vi "NIIE_Settings Init.vi"(7 "Refs":T8, 8 "Error":errorcluster, 10 "Active Tag":string="Icon Editor", 11 "Data In":T1={"Class"={"Ants"=refnum, "Layer"=refnum, "Templates"=refnum, "Icon"=refnum, "Glyph"=refnum, "Settings"=refnum, "Tools"=refnum}, "Ref"={"Add Layer"=refnum, "Remove Layer"=refnum, "Line Text"=[], "Body Text Spec"=refnum, "DNL_Font"=refnum, "glyph path str"=refnum, "templates path str"=refnum, "Arrow Up"=refnum, "Arrow Down"=refnum, "IE VI Ref"=refnum, "Glyphs tree"=refnum, "Templates tree"=refnum, "Layer Icon Text"=refnum, "Layer Template"=refnum, "Clipboard"=refnum, "BW icon in"=refnum, "Color icon in"=refnum, "Layer Clust"=refnum, "Body Text"=refnum, "DNL_Framework Templates"=refnum, "Search Templates"=refnum, "TextMarker"=refnum, "Tab Control"=refnum, "Search Glyphs"=refnum, "Line Color"=refnum, "DNL_Glyphs []"=refnum, "Fill Color"=refnum, "Tools"=refnum, "Glyphs tree"=refnum, "Icon"=refnum, "Preview"=refnum, "Ants"=refnum, "Terminals"=refnum, "menu reference"=refnum, "LayerNames"=[], "GlyphLoadAnimation"=refnum, "TemplateLoadAnimation"=refnum, "refreshGlyphs"=refnum, "refreshTemplates"=refnum}, "Support"={"AntsRect"={"left"=0, "top"=0, "right"=0, "bottom"=0}, "Mouse Move Coords"={"Horizontal"=0, "Vertical"=0}, "Mouse Down Coords"={"Horizontal"=0, "Vertical"=0}, "Temp Coord"={"Horizontal"=0, "Vertical"=0}, "Action"=enum."Default", "Edge Color"=4914962, "Fill Color"=16860, "Mouse Down?"=FALSE, "Draft Mode?"=FALSE, "Temp Icon"=bytes[3102], "CTRL Pressed"=FALSE, "Move Selection?"=FALSE, "AntsRect Orig"={"left"=0, "top"=0, "right"=0, "bottom"=0}, "Text"="", "TM Set?"=FALSE, "Mouse inside icon?"=FALSE, "Tool (old value)"=0, "Pencil Move Color"=0, "Swap Colors?"=FALSE, "Shift pressed?"=FALSE}}) -> (0 "Error Out":errorcluster, 3 "Data In Out":T1={"Class"={"Ants"=refnum, "Layer"=refnum, "Templates"=refnum, "Icon"=refnum, "Glyph"=refnum, "Settings"=refnum, "Tools"=refnum}, "Ref"={"Add Layer"=refnum, "Remove Layer"=refnum, "Line Text"=[], "Body Text Spec"=refnum, "DNL_Font"=refnum, "glyph path str"=refnum, "templates path str"=refnum, "Arrow Up"=refnum, "Arrow Down"=refnum, "IE VI Ref"=refnum, "Glyphs tree"=refnum, "Templates tree"=refnum, "Layer Icon Text"=refnum, "Layer Template"=refnum, "Clipboard"=refnum, "BW icon in"=refnum, "Color icon in"=refnum, "Layer Clust"=refnum, "Body Text"=refnum, "DNL_Framework Templates"=refnum, "Search Templates"=refnum, "TextMarker"=refnum, "Tab Control"=refnum, "Search Glyphs"=refnum, "Line Color"=refnum, "DNL_Glyphs []"=refnum, "Fill Color"=refnum, "Tools"=refnum, "Glyphs tree"=refnum, "Icon"=refnum, "Preview"=refnum, "Ants"=refnum, "Terminals"=refnum, "menu reference"=refnum, "LayerNames"=[], "GlyphLoadAnimation"=refnum, "TemplateLoadAnimation"=refnum, "refreshGlyphs"=refnum, "refreshTemplates"=refnum}, "Support"={"AntsRect"={"left"=0, "top"=0, "right"=0, "bottom"=0}, "Mouse Move Coords"={"Horizontal"=0, "Vertical"=0}, "Mouse Down Coords"={"Horizontal"=0, "Vertical"=0}, "Temp Coord"={"Horizontal"=0, "Vertical"=0}, "Action"=enum."Default", "Edge Color"=4914962, "Fill Color"=16860, "Mouse Down?"=FALSE, "Draft Mode?"=FALSE, "Temp Icon"=bytes[3102], "CTRL Pressed"=FALSE, "Move Selection?"=FALSE, "AntsRect Orig"={"left"=0, "top"=0, "right"=0, "bottom"=0}, "Text"="", "TM Set?"=FALSE, "Mouse inside icon?"=FALSE, "Tool (old value)"=0, "Pencil Move Color"=0, "Swap Colors?"=FALSE, "Shift pressed?"=FALSE}})   [LabVIEW 2021]
uses:
  Controls/Settings.ctl
  Controls/IE Data.ctl
  Class/Ants/Ants.lvclass
  Class/FakedArray/FakedArray.lvclass
  Class/Icon Library/Glyph.lvclass
  Class/Settings/Settings.lvclass
  Class/Tools/Tools Paint.lvclass
  vi.lib/LabVIEW Icon API/lv_icon/Classes/Icon/Icon.lvclass
  Controls/IE Classes.ctl
  Controls/References Cluster.ctl
  Controls/SupportClass.ctl
  <vilib>/Utility/miscctls.llb/LVPoint32TypeDef.ctl
  Controls/ENUM_SupportClass_Action.ctl
  vi.lib/LabVIEW Icon API/lv_icon/Controls/IEColor.ctl
  vi.lib/LabVIEW Icon API/lv_icon/Controls/Pathes.ctl
  vi.lib/LabVIEW Icon API/lv_icon/lv_icon.lvlib
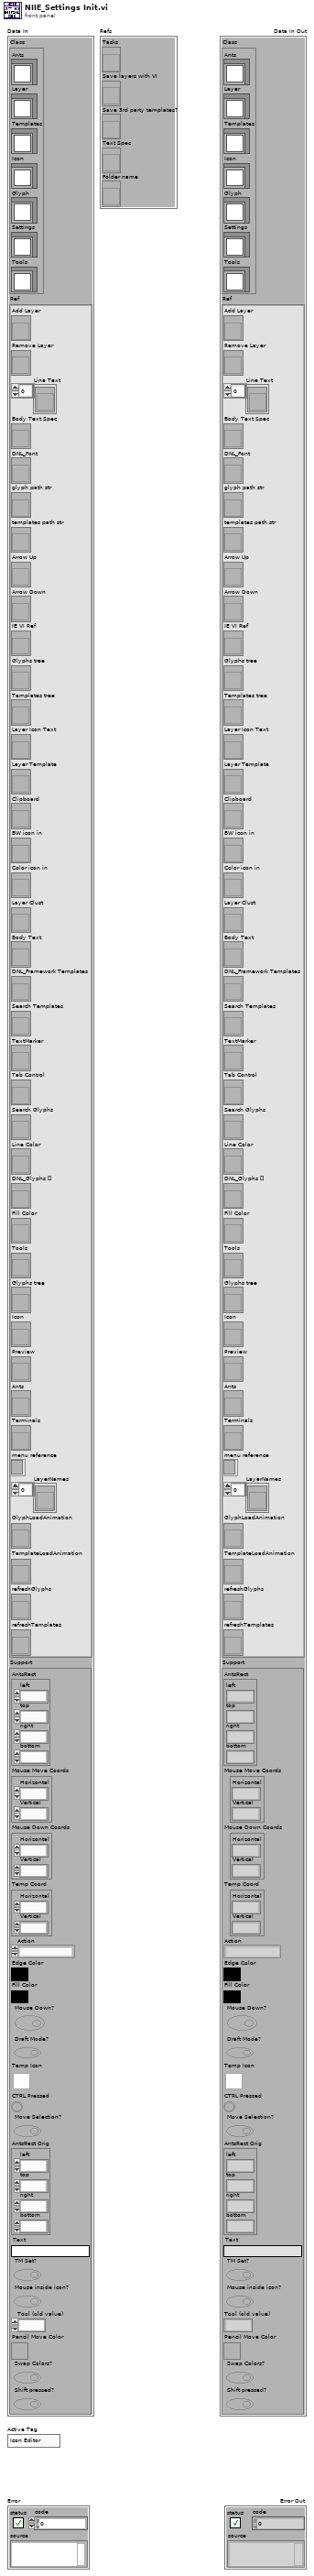
[diagram p1: front panel]
types:
  T1 = typedef "IE Data.ctl" = cluster{"Class":T2, "Ref":T3, "Support":T4}
  T2 = typedef "IE Classes.ctl" = cluster{"Ants":refnum<class "Ants.lvclass">, "Layer":refnum<class "FakedArray.lvclass">, "Templates":refnum<class "FakedArray.lvclass">, "Icon":refnum<class "Icon.lvclass">, "Glyph":refnum<class "Glyph.lvclass">, "Settings":refnum<class "Settings.lvclass">, "Tools":refnum<class "Tools Paint.lvclass">}
  T3 = typedef "References Cluster.ctl" = cluster{"Add Layer":refnum<vi>, "Remove Layer":refnum<vi>, "Line Text":refnum<vi>[], "Body Text Spec":refnum<vi>, "DNL_Font":refnum<vi>, "glyph path str":refnum<vi>, "templates path str":refnum<vi>, "Arrow Up":refnum<vi>, "Arrow Down":refnum<vi>, "IE VI Ref":refnum<vi>, "Glyphs tree":refnum<vi>, "Templates tree":refnum<vi>, "Layer Icon Text":refnum<vi>, "Layer Template":refnum<vi>, "Clipboard":refnum<vi>, "BW icon in":refnum<vi>, "Color icon in":refnum<vi>, "Layer Clust":refnum<vi>, "Body Text":refnum<vi>, "DNL_Framework Templates":refnum<vi>, "Search Templates":refnum<vi>, "TextMarker":refnum<vi>, "Tab Control":refnum<vi>, "Search Glyphs":refnum<vi>, "Line Color":refnum<vi>, "DNL_Glyphs []":refnum<vi>, "Fill Color":refnum<vi>, "Tools":refnum<vi>, "Glyphs tree":refnum<vi>, "Icon":refnum<vi>, "Preview":refnum<vi>, "Ants":refnum<vi>, "Terminals":refnum<vi>, "menu reference":refnum<k9>, "LayerNames":refnum<vi>[], "GlyphLoadAnimation":refnum<vi>, "TemplateLoadAnimation":refnum<vi>, "refreshGlyphs":refnum<vi>, "refreshTemplates":refnum<vi>}
  T4 = typedef "SupportClass.ctl" = cluster{"AntsRect":cluster{"left":i16, "top":i16, "right":i16, "bottom":i16}, "Mouse Move Coords":T5, "Mouse Down Coords":T5, "Temp Coord":T5, "Action":T6, "Edge Color":T7, "Fill Color":T7, "Mouse Down?":bool, "Draft Mode?":bool, "Temp Icon":picture, "CTRL Pressed":bool, "Move Selection?":bool, "AntsRect Orig":cluster{"left":i16, "top":i16, "right":i16, "bottom":i16}, "Text":string, "TM Set?":bool, "Mouse inside icon?":bool, "Tool (old value)":u32, "Pencil Move Color":u32, "Swap Colors?":bool, "Shift pressed?":bool}
  T5 = typedef "LVPoint32TypeDef.ctl" = cluster{"Horizontal":i32, "Vertical":i32}
  T6 = typedef "ENUM_SupportClass_Action.ctl" = enum16{"Default", "Move Selection", "Glyph Library", "Tool"}
  T7 = typedef "IEColor.ctl" = u32
  T8 = typedef "Settings.ctl" = cluster{"Tasks":refnum<vi>, "Save layers with VI":refnum<vi>, "Save 3rd party templates?":refnum<vi>, "Text Spec":refnum<vi>, "Folder name":refnum<vi>}
  T9 = typedef "Pathes.ctl" = enum16{"Root Path", "Icon Templates", "Icon Templates VI", "Icon Templates Lib", "Glyphs"}
  T10 = typedef "Font.ctl" = string
  T11 = typedef "Alignment.ctl" = u16
  T12 = typedef "Num_Font Size.ctl" = u8
  T13 = cluster{"Same Folder Structure?":bool, "Folder Name":string}
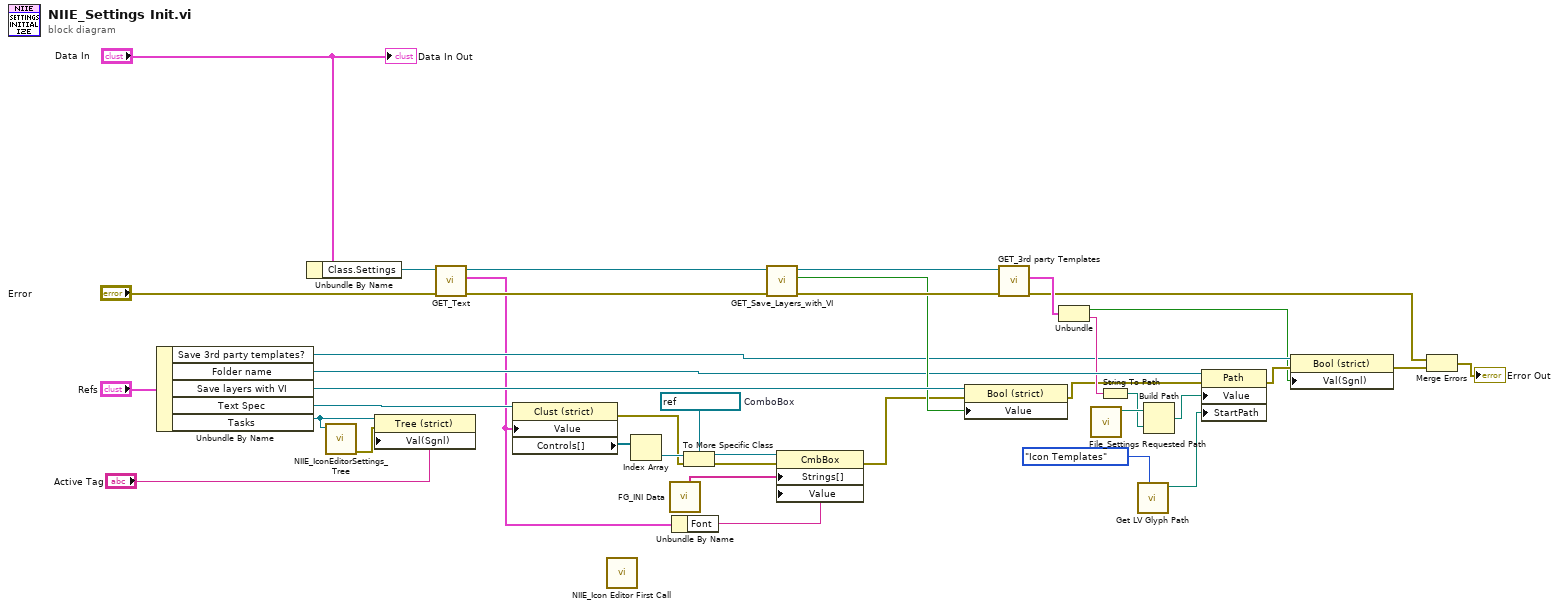
[diagram p0: block diagram]
diagram:
  w15 = refnum<vi> refnum  # ComboBox
  n1 = Unbundle By Name("Refs") -> ("Save 3rd party templates?"=w27:refnum<vi>, "Folder name"=w30:refnum<vi>, "Save layers with VI"=w33:refnum<vi>, "Text Spec"=w34:refnum<vi>, "Tasks"=w2:refnum<vi>)
  n2 = Unbundle By Name("Data In") -> ("Class.Settings"=w12:refnum<class "Settings.lvclass">)
  n3 = call "NIIE_IconEditorSettings_Tree.vi"("Tree Refnum"=w2) -> ("Error Out"=w1:errorcluster)  [unwired: 10 in]
  n4 = property class="Tree (strict)"(reference=w2, error in=w1, "Val(Sgnl)"="Active Tag") -> ()  [unwired: 2 out]
  n5 = call-dynamic "GET_Text.vi"("error in (no error)"="Error", "Settings.lvclass in"=w12) -> ("error out"=w37:errorcluster, "Text"=w14:cluster{"Font":T10, "Alignment":T11, "Size":T12}, "Settings.lvclass out"=w36:refnum<class "Settings.lvclass">)  [unwired: 7 out]
  n6 = property class="Clust (strict)"(reference=w34, "Value"=w14) -> (error out=w16:errorcluster, "Controls[]"=w18:refnum<vi>[])  [unwired: 1 in, 1 out]
  n7 = call "NIIE_Icon Editor First Call.vi"() -> ()  [unwired: 1 in, 11 out]
  n8 = Index Array(array=w18) -> (element=w17:refnum<vi>)  [unwired: 1 in]
  n9 = call "FG_INI Data.vi"() -> ("Font List Out"=w8:string[])  [unwired: 9 in, 2 out]
  n10 = Unbundle By Name(w14) -> ("Font"=w7:T10)
  n11 = To More Specific Class(target class=w15, reference=w17, error in=w16) -> (specific class reference=w6:refnum<vi>, error out=w5:errorcluster)
  n12 = call "GET_Save_Layers_with_VI.vi"("error in (no error)"=w37, "Settings.lvclass in"=w36) -> ("error out"=w38:errorcluster, "Merge user layers on commit"=w32:bool, "Settings.lvclass out"=w39:refnum<class "Settings.lvclass">)  [unwired: 7 out]
  n13 = property class="CmbBox"(reference=w6, error in=w5, "Strings[]"=w8, "Value"=w7) -> (error out=w4:errorcluster)  [unwired: 1 out]
  n14 = property class="Bool (strict)"(reference=w33, error in=w4, "Value"=w32) -> (error out=w28:errorcluster)  [unwired: 1 out]
  n15 = call-dynamic "GET_3rd party Templates.vi"("error in (no error)"=w38, "Settings.lvclass in"=w39) -> ("error out"=w11:errorcluster, "3rd party Templates"=w31:T13)  [unwired: 8 out]
  n16 = Unbundle(w31) -> ("Same Folder Structure?"=w25:bool, "Folder Name"=w29:string)
  n17 = call "File_Settings Requested Path.vi"() -> ("Requested Path"=w21:path)  [unwired: 11 out]
  n18 = String To Path(string=w29) -> (path=w20:path)
  n19 = call "Get LV Glyph Path.vi"("Path"=Pathes."Icon Templates") -> ("Requested Path"=w22:path)  [unwired: 2 in, 8 out]
  n20 = Build Path(base path=w21, name or relative path=w20) -> (appended path=w19:path)
  n21 = property class="Path"(reference=w30, error in=w28, "Value"=w19, "StartPath"=w22) -> (error out=w26:errorcluster)  [unwired: 1 out]
  n22 = property class="Bool (strict)"(reference=w27, error in=w26, "Val(Sgnl)"=w25) -> (error out=w10:errorcluster)  [unwired: 1 out]
  n23 = Merge Errors(w11, w10) -> (→"Error Out":errorcluster)
  "Data In Out" <- "Data In"
